vi "Set Timer.vi"(10 "Max Time (-1ms)":i32, 11 "DMM Driver in":refnum<class "DMM Driver.lvclass">) -> (3 "DMM Driver out":refnum<class "DMM Driver.lvclass">)   [LabVIEW 2020, in "DMM.lvlib" / "DMM Driver.lvclass"]
doc: "Set the measurement timer for the DMM. A value of '-1' disables the timer."
uses:
  DMM Driver.lvclass
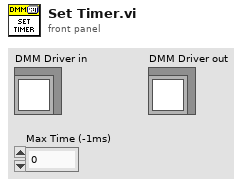
[diagram p1: front panel]
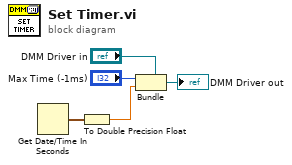
[diagram p0: block diagram]
diagram:
  n1 = Get Date/Time In Seconds() -> (seconds since 1Jan1904=w5:timestamp)
  n2 = To Double Precision Float(number=w5) -> (double precision float=w1:dbl)
  n3 = Bundle(cluster="DMM Driver in", "Max Time (-1ms)", w1) -> (→"DMM Driver out":refnum<class "DMM Driver.lvclass">)
